vi "SuperNS_ParseError.vi"(11 "error in (no error)":errorcluster) -> (15 "error out":errorcluster)   [LabVIEW 2018, in "SuperNS.lvclass"]
doc: "Copyright © 2008 - 2024 VI Technologies B.V. \nALL RIGHTS RESERVED"
uses:
  SuperNS.lvclass
panel:
  # "Copyright (c) 2024, VI Technologies B.V.\nAll rights reserved.\n\nRedistribution and use in source and binary forms, with or without modification, are permitted provided that \nthe following conditions are met:\n\n * Redistributions of source code must retain the above copyright notice, this list of conditions and the \nfollowing disclaimer.\n * Redistributions in binary form must reproduce the above copyright notice, this list of conditions and the \nfollowing disclaimer in the documentation and/or other materials provided with the distribution.\n * Neither the name of VI Technologies B.V. nor the names of its contributors may be used to endorse or \npromote products derived from this software without specific prior written permission.\n\nTHIS SOFTWARE IS PROVIDED BY THE COPYRIGHT HOLDERS AND CONTRIBUTORS \"AS IS\" AND ANY EXPRESS OR \nIMPLIED WARRANTIES, INCLUDING, BUT NOT LIMITED TO, THE IMPLIED WARRANTIES OF MERCHANTABILITY \nAND FITNESS FOR A PARTICULAR PURPOSE ARE DISCLAIMED. IN NO EVENT SHALL THE COPYRIGHT OWNER OR \nCONTRIBUTORS BE LIABLE FOR ANY DIRECT, INDIRECT, INCIDENTAL, SPECIAL, EXEMPLARY, OR CONSEQUENTIAL \nDAMAGES (INCLUDING, BUT NOT LIMITED TO, PROCUREMENT OF SUBSTITUTE GOODS OR SERVICES; LOSS OF \nUSE, DATA, OR PROFITS; OR BUSINESS INTERRUPTION) HOWEVER CAUSED AND ON ANY THEORY OF LIABILITY, \nWHETHER IN CONTRACT, STRICT LIABILITY, OR TORT (INCLUDING NEGLIGENCE OR OTHERWISE) ARISING IN ANY \nWAY OUT OF THE USE OF THIS SOFTWARE, EVEN IF ADVISED OF THE POSSIBILITY OF SUCH DAMAGE.\n\nFor more information, please visit https://www.vi-tech.nl or contact us at info@vi-tech.nl"
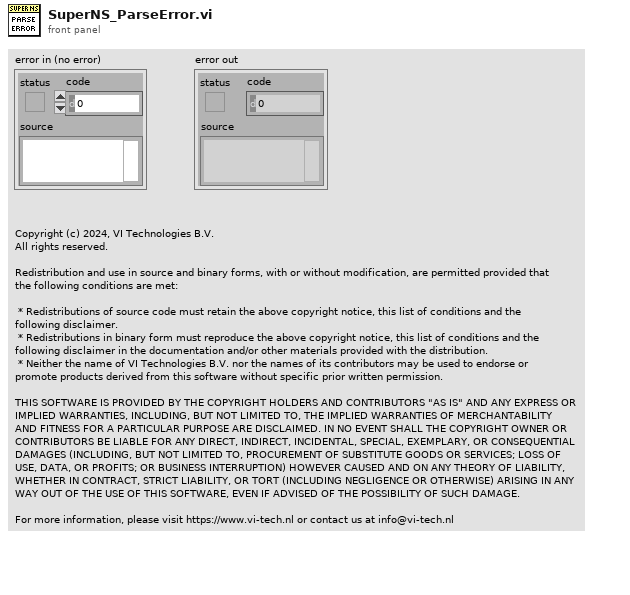
[diagram p1: front panel]
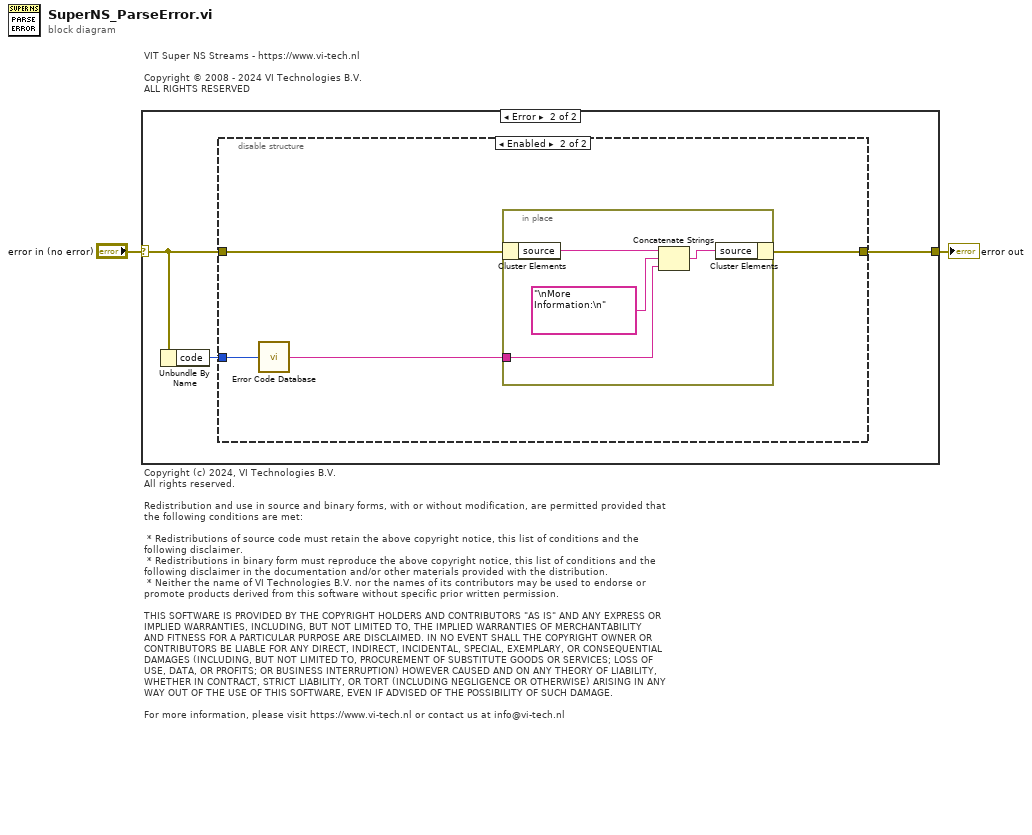
[diagram p0: block diagram]
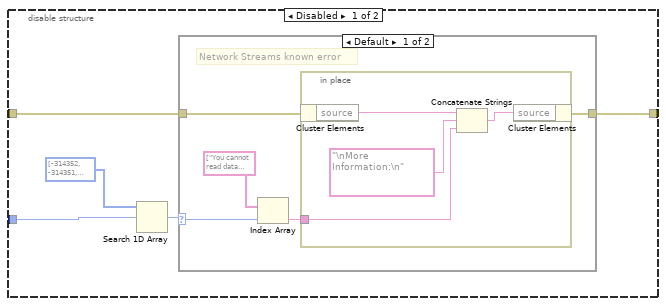
[diagram p3: hidden frame]
diagram:
  # "VIT Super NS Streams - https://www.vi-tech.nl\n\nCopyright © 2008 - 2024 VI Technologies B.V. \nALL RIGHTS RESERVED"
  # "Copyright (c) 2024, VI Technologies B.V.\nAll rights reserved.\n\nRedistribution and use in source and binary forms, with or without modification, are permitted provided that \nthe following conditions are met:\n\n * Redistributions of source code must retain the above copyright notice, this list of conditions and the \nfollowing disclaimer.\n * Redistributions in binary form must reproduce the above copyright notice, this list of conditions and the \nfollowing disclaimer in the documentation and/or other materials provided with the distribution.\n * Neither the name of VI Technologies B.V. nor the names of its contributors may be used to endorse or \npromote products derived from this software without specific prior written permission.\n\nTHIS SOFTWARE IS PROVIDED BY THE COPYRIGHT HOLDERS AND CONTRIBUTORS \"AS IS\" AND ANY EXPRESS OR \nIMPLIED WARRANTIES, INCLUDING, BUT NOT LIMITED TO, THE IMPLIED WARRANTIES OF MERCHANTABILITY \nAND FITNESS FOR A PARTICULAR PURPOSE ARE DISCLAIMED. IN NO EVENT SHALL THE COPYRIGHT OWNER OR \nCONTRIBUTORS BE LIABLE FOR ANY DIRECT, INDIRECT, INCIDENTAL, SPECIAL, EXEMPLARY, OR CONSEQUENTIAL \nDAMAGES (INCLUDING, BUT NOT LIMITED TO, PROCUREMENT OF SUBSTITUTE GOODS OR SERVICES; LOSS OF \nUSE, DATA, OR PROFITS; OR BUSINESS INTERRUPTION) HOWEVER CAUSED AND ON ANY THEORY OF LIABILITY, \nWHETHER IN CONTRACT, STRICT LIABILITY, OR TORT (INCLUDING NEGLIGENCE OR OTHERWISE) ARISING IN ANY \nWAY OUT OF THE USE OF THIS SOFTWARE, EVEN IF ADVISED OF THE POSSIBILITY OF SUCH DAMAGE.\n\nFor more information, please visit https://www.vi-tech.nl or contact us at info@vi-tech.nl"
  n1 = case shown="Error" "error in (no error)" {
    selector: "error in (no error)" -> [w3 w4]
    tunnel: [w3 w5] -> w1
    frame No Error {
    }
    frame Error {
      n2 = Unbundle By Name(w4) -> ("code"=w6:i32)
      n3 = disable-structure shown="Enabled" {
        disable-tunnel: w6 -> [w11 w25]
        disable-tunnel: [w9 w23] -> w5
        disable-tunnel: w4 -> [w8 w24]
        frame Disabled {
          n4 = Search 1D Array(1D array=i32[] [-314352, -314351, -314350, -314340, -314335, -314320, -314310, -314305, -314302, -314246, -314245, -314240, -314235, -314230, -314227, -314226, -314220, -314215, -314202, -314201, -314109, -314108, -314107, -314106, -314105, -314104, -314103, -314102, -314101, -314100, -314054, -314053, -314052, -314051, -314050, -314009, -314008, -314007, -314006, -314005, -314004, -314003, -314002, -314001, -314000, 314000, 314001, 314010, 314050, 314051, 314205, 314210] ("ErrorCodes"), element=w11) -> (index of element=w10:i32)  [unwired: 1 in]
          n5 = case shown="Default" w10 {
            selector: w10 -> [w13 _]
            tunnel: [w15 w21] -> w9
            tunnel: w8 -> [w16 w21]
            frame Default {
              # "Network Streams known error"
              n6 = Index Array(array=string[] ["You cannot read data from a writer endpoint or write data to a reader endpoint. Ensure that you have not wired a Write Single Element to Stream, Write Multiple Elements to Stream, or Flush Stream function to a Create Network Stream Reader Endpoint function. Conversely, ensure that you have not wired a Read Single Element from Stream or Read Multiple Elements from Stream function to a Create Network Stream Writer Endpoint function. ", "You must read or write elements of the same data type that you wired to the data type terminal of the Create Network Stream Reader Endpoint or Create Network Stream Writer Endpoint function. ", "Another application is already streaming data to an endpoint in the context you specified. If you specified a context name in the reader name or writer name terminal of the endpoint, you must specify an unused context name. If you did not specify a context name, you must specify an unused context name by entering an endpoint URL in the reader name or writer name terminal. ", "The local endpoint found the remote endpoint at the URL you specified, but the remote endpoint was trying to connect to a third endpoint. Ensure that corresponding endpoints each specify the URL of the other endpoint, or specify a URL with only one of the endpoints so the other endpoint accepts a connection from the first endpoint that connects to it. ", "The local endpoint was restarted because the computer that hosts the remote endpoint crashed, was rebooted, or experienced a hang. ", "LabVIEW could not create the remote endpoint because the computer that hosts the endpoint ran out of memory. ", "The remote endpoint has been destroyed. ", "The protocol version of the writer endpoint is not compatible with the protocol version of the reader endpoint. To transfer data between these endpoints, you must upgrade the version of LabVIEW that the older endpoint uses. ", "The remote endpoint is already connected to another endpoint. Each endpoint can connect to only one other endpoint at a time. ", "The remote and local endpoints are either both reader endpoints or both writer endpoints. You can prompt a connection between a reader and writer endpoint only . ", "The data type of the remote endpoint does not match the data type of the local endpoint. The data types of the endpoints must match. ", "The stream detected an unrecoverable loss of data. Contact National Instruments for support. ", "The remote endpoint was restarted because the computer that hosts the endpoint crashed, was rebooted, or experienced a hang. ", "LabVIEW could not create the local endpoint because the computer that hosts the endpoint ran out of memory. ", "The URL you specified with the reader url or writer url terminal does not include the name of the remote endpoint. You must specify a valid endpoint URL in one of these terminals to connect two endpoints together. ", "Incompatible format. ", "The remote endpoint has been destroyed. ", "You cannot read or write a number of elements that is larger than the size of the endpoint buffer. ", "You cannot flush a network stream from the reader endpoint. Call the Flush Stream function from the writer endpoint only. ", "The local endpoint lost connection and reconnected with the remote endpoint, but some data was lost. ", "The name of one endpoint cannot be the partial name of another endpoint within the same application. Change the name of this endpoint so that it does not overlap with an existing name, or destroy the other endpoint before creating this endpoint. ", "The name of one endpoint cannot be the partial name of another endpoint within the same application. Change the name of this endpoint so that it does not overlap with an existing name, or destroy the other endpoint before creating this endpoint. ", "The local endpoint is already connected to another endpoint. Each endpoint can connect to only one other endpoint at a time. ", "The local endpoint is not connected to a remote endpoint. Specify the URL of a remote endpoint in the writer url terminal of the Create Network Stream Reader Endpoint function or the reader url terminal of the Create Network Stream Writer Endpoint function to prompt a connection between two endpoints. ", "You can call the Write Single Element to Stream and Write Multiple Elements to Stream functions from the writer endpoint only. ", "You can call the Read Single Element from Stream and Read Multiple Elements from Stream functions from the reader endpoint only. ", "You did not specify an endpoint name. Specify a valid name or endpoint URL with the reader name terminal of the Create Network Stream Reader Endpoint function or the writer name terminal of the Create Network Stream Writer Endpoint function. ", "The buffer size of the endpoint must be greater than zero elements. ", "An endpoint with the same name already exists. ", "The specified endpoint does not exist. ", "The Network Streams Engine cannot be uninitialized. ", "The Network Streams Engine failed to initialize. ", "The Network Streams Engine is not initialized. ", "The Network Streams Engine was already initialized. ", "The Network Streams Engine does not exist. ", "The value wired to the Wait Condition input is invalid. Refer to the LabVIEW Help for valid values. ", "The value wired to the Element Allocation Mode input is invalid. Refer to the LabVIEW Help for valid values. ", "You cannot read multiple array elements of different dimensions. You can read multiple array elements of the same dimension only. ", "You cannot specify a relative URL with the reader url and writer url terminals. You must use an absolute URL instead. For example, if you are connecting to an endpoint with the name Endpoint1 on a computer with the IP address 10.0.0.62, use the URL //10.0.0.62/stream1. ", "The ni_nwstreams library contains invalid parameters. ", "LabVIEW could not create the endpoint within the timeout period. Ensure that you specify the URL of a remote endpoint with the reader url terminal of the Create Network Stream Writer Endpoint function or the writer url terminal of the Create Network Stream Reader Endpoint function. ", "LabVIEW could not create a network stream. You must specify the URL of a remote endpoint with either the reader url terminal of the Create Network Stream Writer Endpoint function or the writer url terminal of the Create Network Stream Reader Endpoint function. ", "You cannot call this property from the reader endpoint. You can call this property from the writer endpoint only. ", "You cannot call this property from the writer endpoint. You can call this property from the reader endpoint only. ", "LabVIEW cannot load the ni_nwstreams library. If you are using a desktop computer, you might need to repair your LabVIEW installation or reinstall LabVIEW or the LabVIEW Run-Time Engine. If you are using an RT target, verify that you installed the network streams feature with Measurement and Automation Explorer (MAX). ", "Not enough elements to read. ", "Not enough free space to write. ", "The writer endpoint was destroyed before it received an acknowledgement from the reader endpoint that all data was received. The reader endpoint might not have received some data. ", "You specified the URL of a remote endpoint that does not exist. ", "The remote endpoint did not prompt a connection with the local endpoint. Make sure you specify the correct URL with the URL terminal of the remote endpoint. ", "The local endpoint did not receive a response from the remote endpoint before the timeout expired. ", "The endpoint timed out before another endpoint prompted a connection with it. "] ("ErrorDescriptions"), index=w13) -> (element=w12:string)
              n7 = in-place {
                in-place-border: w12 -> [w18]
                n8 = in-place-cluster #1(w16) -> ("source"=w20:string)
                n9 = Concatenate Strings(w20, "\nMore Information:\n" ("string"), w18) -> (w17:string)
                n10 = in-place-cluster #1("source"=w17) -> (w15:errorcluster)
              }
            }
            frame -1 {
            }
          }
        }
        frame Enabled {
          n11 = call <vilib>:"Error Code Database.vi"("Error Code"=w25) -> ("Error Text"=w22:string)
          n12 = in-place {
            in-place-border: w22 -> [w27]
            n13 = in-place-cluster #2(w24) -> ("source"=w29:string)
            n14 = Concatenate Strings(w29, "\nMore Information:\n" ("string"), w27) -> (w26:string)
            n15 = in-place-cluster #2("source"=w26) -> (w23:errorcluster)
          }
        }
      }
    }
  }
  "error out" <- w1
